vi "Zeta Modification of Negative Number.vi"(11 "x":cdb) -> (3 "r(x)":cdb)   [LabVIEW 2010, in "NI_Gmath.lvlib"]
uses:
  NI_Gmath.lvlib
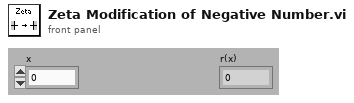
[diagram p1: front panel]
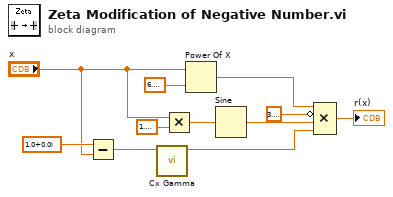
[diagram p0: block diagram]
diagram:
  n1 = Subtract(x=cdb 1.0+0.0i, y="x") -> (x-y=w2:cdb)
  n2 = call "Cx Gamma.vi"("z"=w2) -> ("g(z)"=w1:cdb)  [unwired: 10 out]
  n3 = Multiply(x="x", y=1.5707963267948966) -> (x*y=w6:cdb)
  n4 = Power Of X(1:6.283185307179586, 2:"x") -> (0:w11:cdb)
  n5 = Sine(x=w6) -> (sin(x)=w7:cdb)
  n6 = Compound Arithmetic op=MULTIPLY(w11, invert 3.141592653589793, w7, w1) -> (→"r(x)":cdb)
